vi "Set Voltage.vi"(8 "error in (no error)":errorcluster, 10 "Voltage":dbl, 11 "PS_Sim in":refnum<class "PS_Sim.lvclass">) -> (0 "error out":errorcluster, 3 "PS_Sim out":refnum<class "PS_Sim.lvclass">)   [LabVIEW 2020, in "PS.lvlib" / "PS_Sim.lvclass"]
uses:
  PS_Sim.lvclass
  PS_Sim.lvclass/PS_Sim.ctl
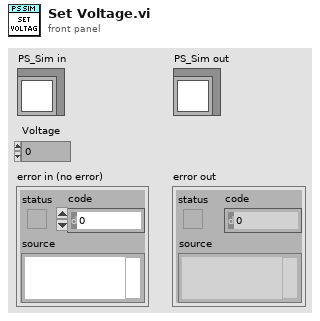
[diagram p1: front panel]
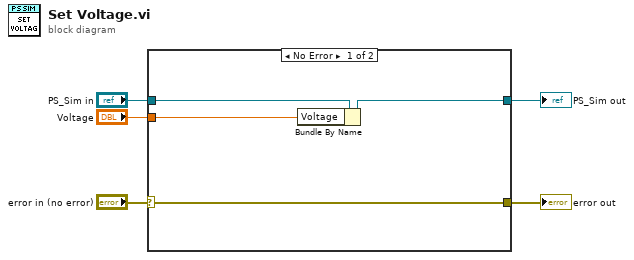
[diagram p0: block diagram]
diagram:
  n1 = case shown="No Error" "error in (no error)" {
    selector: "error in (no error)" -> [w8 w10]
    tunnel: [w7 w11] -> w4
    tunnel: "PS_Sim in" -> [w9 w11]
    tunnel: [w8 w10] -> w2
    tunnel: "Voltage" -> [w6 _]
    frame No Error {
      n2 = Bundle By Name(cluster=w9, "Voltage"=w6) -> (w7:refnum<class "PS_Sim.lvclass">)
    }
    frame Error {
    }
  }
  "error out" <- w2
  "PS_Sim out" <- w4
